vi "Cursor_calc_voltage.vi"(9 "Y":dbl, 10 "X":dbl, 11 "Scan Parameters":T1 {"fill frac" min=0.0 max=1.0 step=0.05; "y voltage max" format="%0.2p"; "y voltage min" format="%0.2p"; "x voltage max" format="%0.2p"; "x voltage min" format="%0.2p"}) -> (2 "Y (Volts)":dbl, 3 "X (Volts)":dbl)   [LabVIEW 2012]
uses:
  typedefs/Scan Parameters.ctl
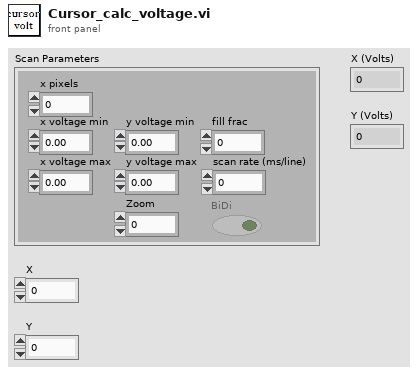
[diagram p1: front panel]
types:
  T1 = typedef "Scan Parameters.ctl" = cluster{"x pixels":i32, "x voltage min":dbl, "x voltage max":dbl, "y voltage min":dbl, "y voltage max":dbl, "fill frac":dbl, "Zoom":dbl, "BiDi":bool, "scan rate (ms/line)":dbl}
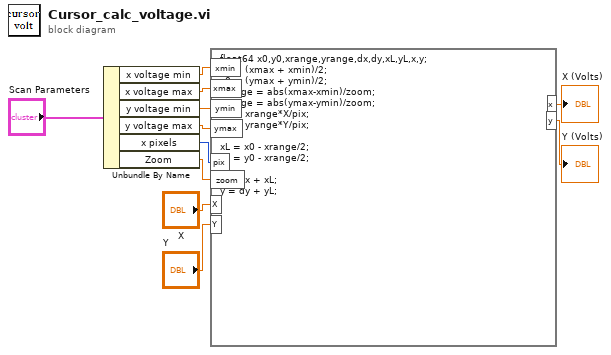
[diagram p0: block diagram]
diagram:
  n1 = Unbundle By Name("Scan Parameters") -> ("x voltage min"=w2:dbl, "x voltage max"=w3:dbl, "y voltage min"=w4:dbl, "y voltage max"=w5:dbl, "x pixels"=w7:i32, "Zoom"=w1:dbl)
  n2 = formula code="float64 x0,y0,xrange,yrange,dx,dy,xL,yL,x,y;\nx0 = (xmax + xmin)/2;\ny0 = (ymax + ymin)/2;\nxrange = abs(xmax-xmin)/zoom;\nyrange = abs(ymax-ymin)/zoom;\ndx = xrange*X/pix;\ndy = yrange*Y/pix;\n\nxL = x0 - xrange/2;\nyL = y0 - xrange/2;\n\nx = dx + xL;\ny = dy + yL;"("xmin"=w2, "xmax"=w3, "ymin"=w4, "ymax"=w5, "X"="X", "Y"="Y", "pix"=w7, "zoom"=w1) -> ("x"=→"X (Volts)":dbl, "y"=→"Y (Volts)":dbl)
